vi "online_status_of_target.vi"(8 "error in (no error)":errorcluster, 10 "String":string) -> (0 "error out":errorcluster, 2 "x >= 0?":bool)   [LabVIEW 2015]
panel:
  out "offset past match":i32
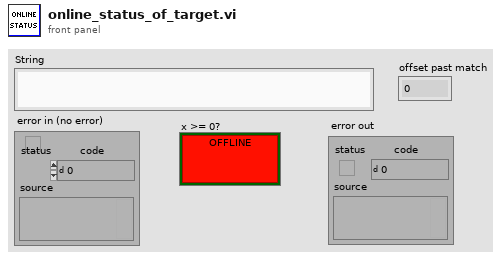
[diagram p1: front panel]
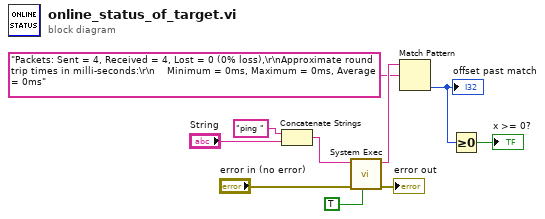
[diagram p0: block diagram]
diagram:
  n1 = Concatenate Strings("ping " ("command line"), "String") -> (w8:string)
  n2 = call <vilib>:"System Exec.vi"("run minimized? (F)"=TRUE, "error in (no error)"="error in (no error)", "command line"=w8) -> ("error out"=→"error out":errorcluster, "standard output"=w4:string)  [unwired: 5 in, 2 out]
  n3 = Match Pattern(string=w4, regular expression="Packets: Sent = 4, Received = 4, Lost = 0 (0% loss),\r\nApproximate round trip times in milli-seconds:\r\n    Minimum = 0ms, Maximum = 0ms, Average = 0ms") -> (offset past match=w2:i32)  [unwired: 1 in, 3 out]
  "offset past match" <- w2
  n4 = Greater Or Equal To 0?(x=w2) -> (x >= 0?=→"x >= 0?":bool)
